vi "Unflatten.vi"(8 "error in (no error)":errorcluster, 9 "Path":path, 11 "Dummy Scan in":refnum<class "Dummy Scan.lvclass">) -> (0 "error out":errorcluster, 3 "Dummy Scan out":refnum<class "Dummy Scan.lvclass">)   [LabVIEW 2009, in "Dummy Scan.lvclass"]
uses:
  Dummy Scan.lvclass
  Scanner/Scanner.lvclass
  <vilib>/Utility/xml.llb/Read From XML File(string).vi
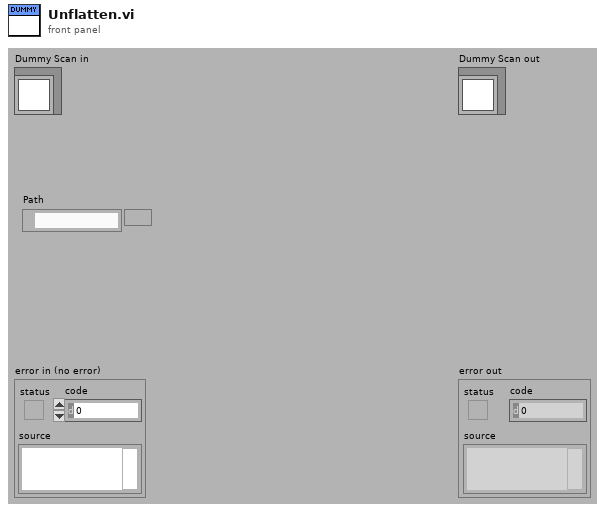
[diagram p1: front panel]
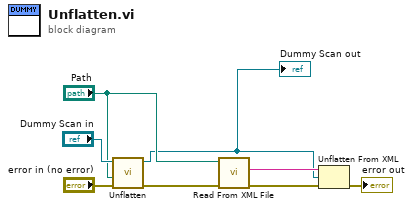
[diagram p0: block diagram]
diagram:
  n1 = call-parent "Unflatten.vi"("error in (no error)"="error in (no error)", "Path"="Path", "Scanner in"="Dummy Scan in") -> ("error out"=w5:errorcluster, "Scanner out"=w1:refnum<class "Dummy Scan.lvclass">)  [unwired: 7 in]
  "Dummy Scan out" <- w1
  n2 = call-poly <vilib>:"Read From XML File.vi"("error in (no error)"=w5, "XML File Path"="Path") -> ("error out"=w6:errorcluster, "XML Elements"=w3:string)  [unwired: 7 in, 1 out]
  n3 = Unflatten From XML(xml string=w3, type=w1, error in (no error)=w6) -> (error out=→"error out":errorcluster)  [unwired: 1 out]
